vi "1-11.vi"() -> ()   [LabVIEW 2022 SP3]
panel:
  in  "单位选择":bool
  out "数值":dbl
  out "温度计":dbl(slide) scale=0.0..100.0
  # "OFF"
  # "摄氏温度"
  # "华氏温度"
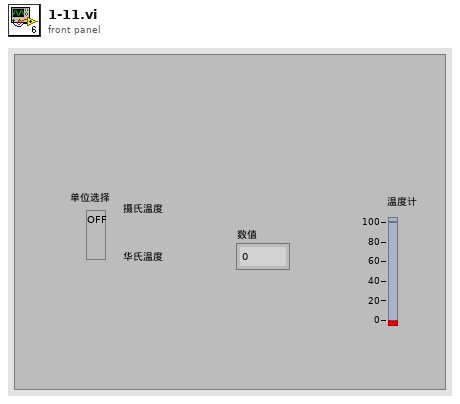
[diagram p1: front panel]
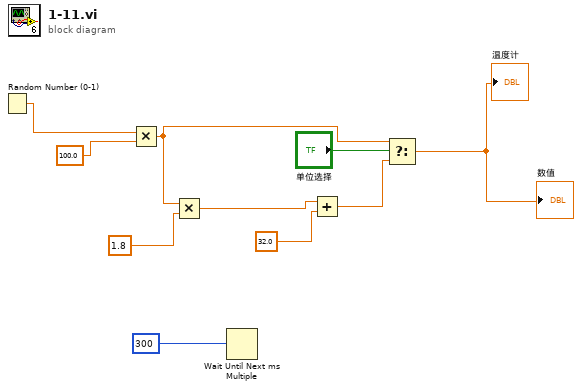
[diagram p0: block diagram]
diagram:
  n1 = Random Number (0-1)() -> (number: 0 to 1=w10:dbl)
  n2 = Multiply(x=w10, y=100.0 ("x*y")) -> (x*y=w7:dbl)
  n3 = Multiply(x=w7, y=1.8 ("x*y")) -> (x*y=w6:dbl)
  n4 = Wait Until Next ms Multiple(millisecond multiple=300) -> ()  [unwired: 1 out]
  n5 = Add(x=w6, y=32.0 ("x")) -> (x+y=w4:dbl)
  n6 = Select(t=w7, s="单位选择", f=w4) -> (s? t:f=→"温度计" →"数值":dbl)
